vi "Test 4.vi"(8 "error in (no error)":errorcluster, 11 "Test Case In":refnum<class "Tests.lvclass">) -> (0 "error out":errorcluster, 3 "Test Case Out":refnum<class "Tests.lvclass">)   [LabVIEW 2021, in "Tests.lvclass"]
uses:
  Tests.lvclass
  C:/Program Files (x86)/National Instruments/LabVIEW 2021/vi.lib/Astemes/LUnit/Test Case.lvclass
  <vilib>/Astemes/LUnit/Test Case.lvclass/Test Case.ctl
  4993e8ee-a06a-463a-9684-69129f64d5ce.vi
  edd98eef-76eb-44a5-86a1-b5d8b1cbf7a6.vi
  <vilib>/Astemes/LUnit/Append Pass Result.vi
  <vilib>/Astemes/LUnit/Append Fail Result.vi
  <vilib>/Astemes/LUnit/Compare Variants.vi
  <vilib>/Astemes/LUnit/Describe Comparison of Arrays.vi
  <vilib>/Astemes/LUnit/Describe Comparison.vi
  <vilib>/Astemes/LUnit/Variant to string.vi
  <vilib>/AdvancedString/1D String Array to Delimited String.vi
  <vilib>/Utility/Data Type/Get Type Information.vi
  <vilib>/Utility/LVClass/Get LV Class Name.vi
  Proto/Module.lvclass
  Tests.lvclass/Tests.ctl
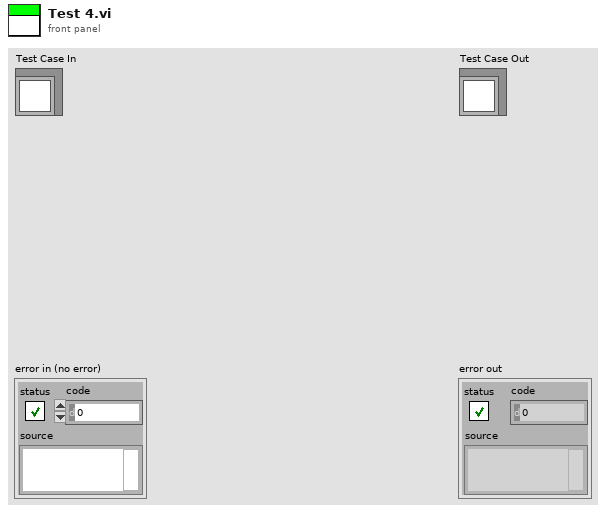
[diagram p1: front panel]
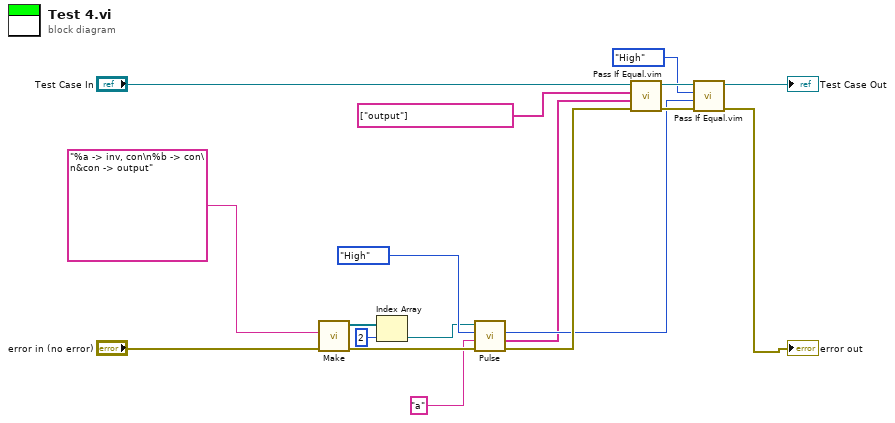
[diagram p0: block diagram]
diagram:
  n1 = call "Make.vi"("error in (no error)"="error in (no error)", "Input"="%a -> inv, con\n%b -> con\n&con -> output") -> ("error out"=w15:errorcluster, "Proto"=w13:refnum<class "Module.lvclass">[])  [unwired: 8 in]
  n2 = Index Array(array=w13, index=2) -> (element=w5:refnum<class "Module.lvclass">)
  n3 = call-dynamic "Pulse.vi"("error in (no error)"=w15, "Sender"="a", "Pulse In"=enum16{"Low", "High"}."High", "Module In"=w5) -> ("error out"=w14:errorcluster, "Receivers"=w1:string[], "Pulse Out"=w2:enum16{"Low", "High"})  [unwired: 4 in, 1 out]
  n4 = call "Pass If Equal.vim"("error in (no error)"=w14, "Actual"=w1, "Expected"=string[] ["output"] ("Receivers"), "LUnit Test Case In"="Test Case In") -> ("error out"=w16:errorcluster, "LUnit Test Case Out"=w9:refnum<class "Tests.lvclass">)  [unwired: 6 in]
  n5 = call "Pass If Equal.vim"("error in (no error)"=w16, "Actual"=w2, "Expected"=enum16{"Low", "High"}."High" ("Pulse In"), "LUnit Test Case In"=w9) -> ("error out"=→"error out":errorcluster, "LUnit Test Case Out"=→"Test Case Out":refnum<class "Tests.lvclass">)  [unwired: 6 in]
